vi "Get Result.vi"(4 "Controller name":string, 6 "Last request":bool, 8 "error in (no error)":errorcluster, 11 "Combined Measurement in":refnum<class "Combined Measurement.lvclass">) -> (0 "error out":errorcluster, 2 "Result":refnum<class "Acquired Result.lvclass">, 3 "Combined Measurement out":refnum<class "Combined Measurement.lvclass">)   [LabVIEW 2021, in "Combined Measurement.lvclass"]
uses:
  Combined Measurement.lvclass
  NHMFL_Core/Libraries/Instruments/Results/Acquired Result/Acquired Result.lvclass
  NHMFL_Core/Libraries/Instruments/Results/Combined Result/Combined Result.lvclass
  C:/Git/NHMFL_Core/Libraries/Instruments/Results/Acquired Result/Acquired Result.lvclass
  NHMFL_Core/Libraries/Instruments/Results/Acquired Result/Acquired Result.lvclass/Acquired Result.ctl
  NHMFL_Core/Libraries/Instruments/Results/Acquired Result/Write Group.vi
  Continuous Recorder Actor/Continuous Recorder Actor.lvclass
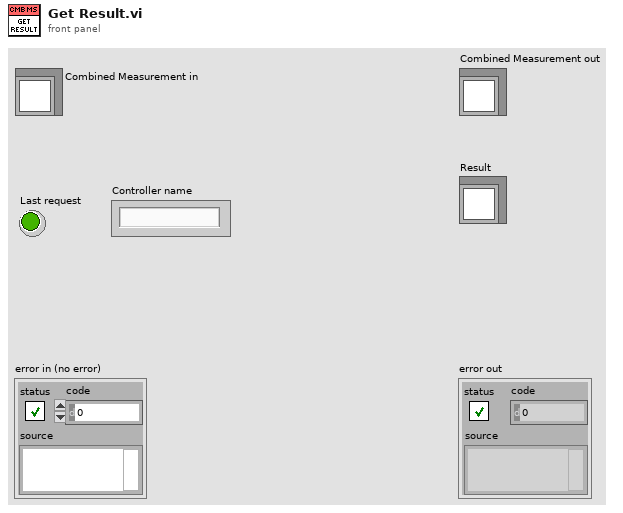
[diagram p1: front panel]
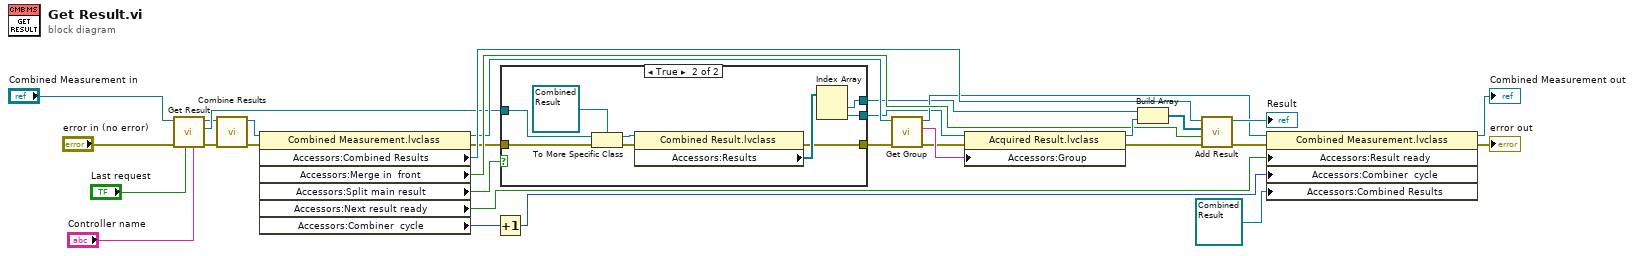
[diagram p0: block diagram]
diagram:
  n1 = call-parent "Get Result.vi"("Controller name"="Controller name", "Last request"="Last request", "error in (no error)"="error in (no error)", "Instrument Recorder in"="Combined Measurement in") -> ("error out"=w3:errorcluster, "Result"=w13:refnum<class "Acquired Result.lvclass">, "Instrument Recorder out"=w4:refnum<class "Combined Measurement.lvclass">)  [unwired: 5 in]
  n2 = call-dynamic "Combine Results.vi"("error in (no error)"=w3, "Combined Measurement in"=w4) -> ("error out"=w2:errorcluster, "Combined Measurement out"=w1:refnum<class "Combined Measurement.lvclass">)  [unwired: 8 in]
  n3 = property class="Combined Measurement.lvclass"(reference=w1, error in=w2) -> (reference out=w17:refnum<class "Combined Measurement.lvclass">, error out=w10:errorcluster, "Accessors:Combined Results"=w27:refnum<class "Combined Result.lvclass">, "Accessors:Merge in  front"=w22:bool, "Accessors:Split main result"=w18:bool, "Accessors:Next result ready"=w6:bool, "Accessors:Combiner  cycle"=w7:i32)
  n4 = Increment(x=w7) -> (x+1=w8:i32)
  n5 = case shown="True" w18 {
    tunnel: w13 -> [w33 w41]
    tunnel: w10 -> [w32 w40]
    tunnel: [w33 w36] -> w14
    tunnel: [w33 w35] -> w12
    tunnel: [w32 w34] -> w11
    frame False {
    }
    frame True {
      n6 = To More Specific Class(target class=refnum<class "Combined Result.lvclass"> refnum ("Combined Result out"), reference=w41, error in=w40) -> (specific class reference=w38:refnum<class "Combined Result.lvclass">, error out=w39:errorcluster)
      n7 = property class="Combined Result.lvclass"(reference=w38, error in=w39) -> (error out=w34:errorcluster, "Accessors:Results"=w37:refnum<class "Acquired Result.lvclass">[])  [unwired: 1 out]
      n8 = Index Array(array=w37) -> (element #1=w35:refnum<class "Acquired Result.lvclass">, element #2=w36:refnum<class "Acquired Result.lvclass">)  [unwired: 2 in]
    }
  }
  n9 = call-dynamic "Get Group.vi"("error in (no error)"=w11, "Combined Measurement in"=w17) -> ("error out"=w9:errorcluster, "Group"=w15:string, "Combined Measurement out"=w16:refnum<class "Combined Measurement.lvclass">)  [unwired: 7 in]
  n10 = property class="Acquired Result.lvclass"(reference=w14, error in=w9, "Accessors:Group"=w15) -> (reference out=w26:refnum<class "Acquired Result.lvclass">, error out=w24:errorcluster)
  n11 = Build Array(w12, w26) -> (w25:refnum<class "Acquired Result.lvclass">[])
  n12 = call-dynamic "Add Result.vi"("error in (no error)"=w24, "Add in front"=w22, "Results to add"=w25, "Combined Result in"=w27) -> ("error out"=w23:errorcluster, "Combined Result out"=→"Result":refnum<class "Combined Result.lvclass">)  [unwired: 6 in]
  n13 = property class="Combined Measurement.lvclass"(reference=w16, error in=w23, "Accessors:Result ready"=w6, "Accessors:Combiner  cycle"=w8, "Accessors:Combined Results"=refnum<class "Combined Result.lvclass"> refnum ("Combined Results")) -> (reference out=→"Combined Measurement out":refnum<class "Combined Measurement.lvclass">, error out=→"error out":errorcluster)
